vi "AmmeterComm.vi"() -> ()   [LabVIEW 2010]
uses:
  VarableID.ctl
  AmmeterGlobalCostants.vi
panel:
  out "display":T1={"电压/V"=[220.633378, 0.0, 0.0, 0.0, 0.0, 0.0, 0.0, 0.0], "测量变量显示"={"number: 0 to 1"=0.0, "number: 0 to 1"=0.0, "number: 0 to 1"=0.0}, "测量变量显示 2"={"number: 0 to 1"=0.0, "number: 0 to 1"=0.0, "number: 0 to 1"=0.0}}
  in  "视在功率":bool=TRUE
  in  "功率因数":bool=TRUE
  in  "电压":bool=TRUE
  in  "电流":bool=TRUE
  in  "退出系统":bool
  in  "软件使用说明":bool
  in  "启动采集":bool=TRUE
  # "CPES能源信息采集系统"
  # "信号采集选项"
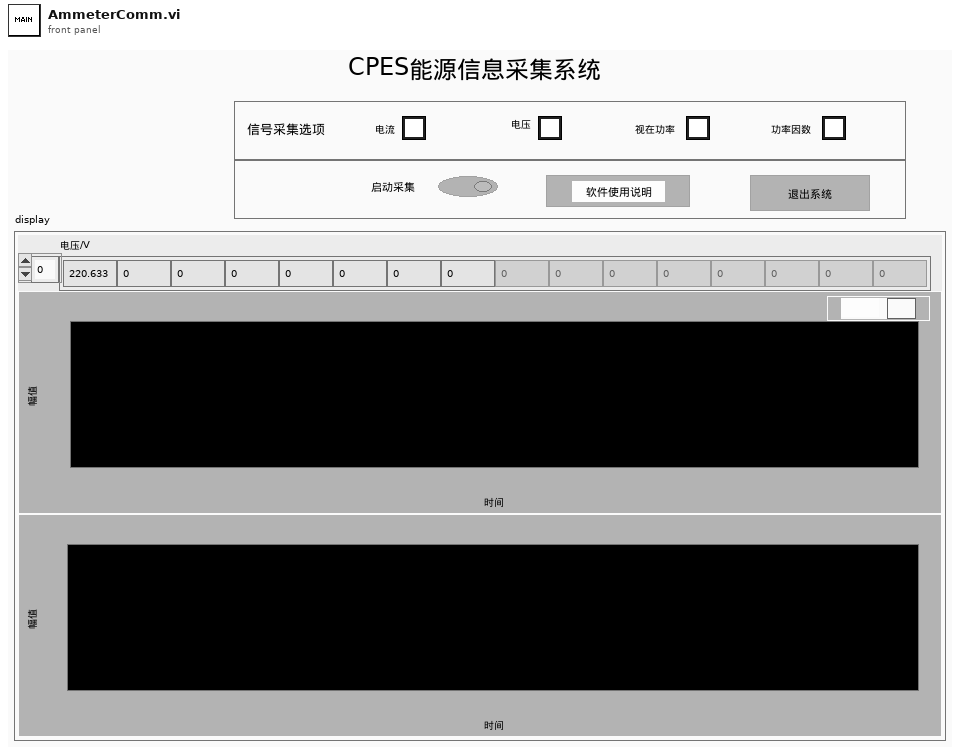
[diagram p1: front panel]
types:
  T1 = cluster{"电压/V":dbl[], "测量变量显示":cluster{"number: 0 to 1":dbl, "number: 0 to 1":dbl, "number: 0 to 1":dbl}, "测量变量显示 2":cluster{"number: 0 to 1":dbl, "number: 0 to 1":dbl, "number: 0 to 1":dbl}}
  T2 = cluster{"测量变量显示":refnum<vi>, "测量变量显示 2":refnum<vi>, "电压/V":refnum<vi>}
  T3 = typedef "OutputDataFormat.ctl" = cluster{"property":string, "dataIdentity":string, "value":string, "address":string, "timeStamp":string, "unit":string, "numID":i32, "VarableID":T4}
  T4 = typedef "VarableID.ctl" = enum16{"current", "power", "PF", "voltage"}
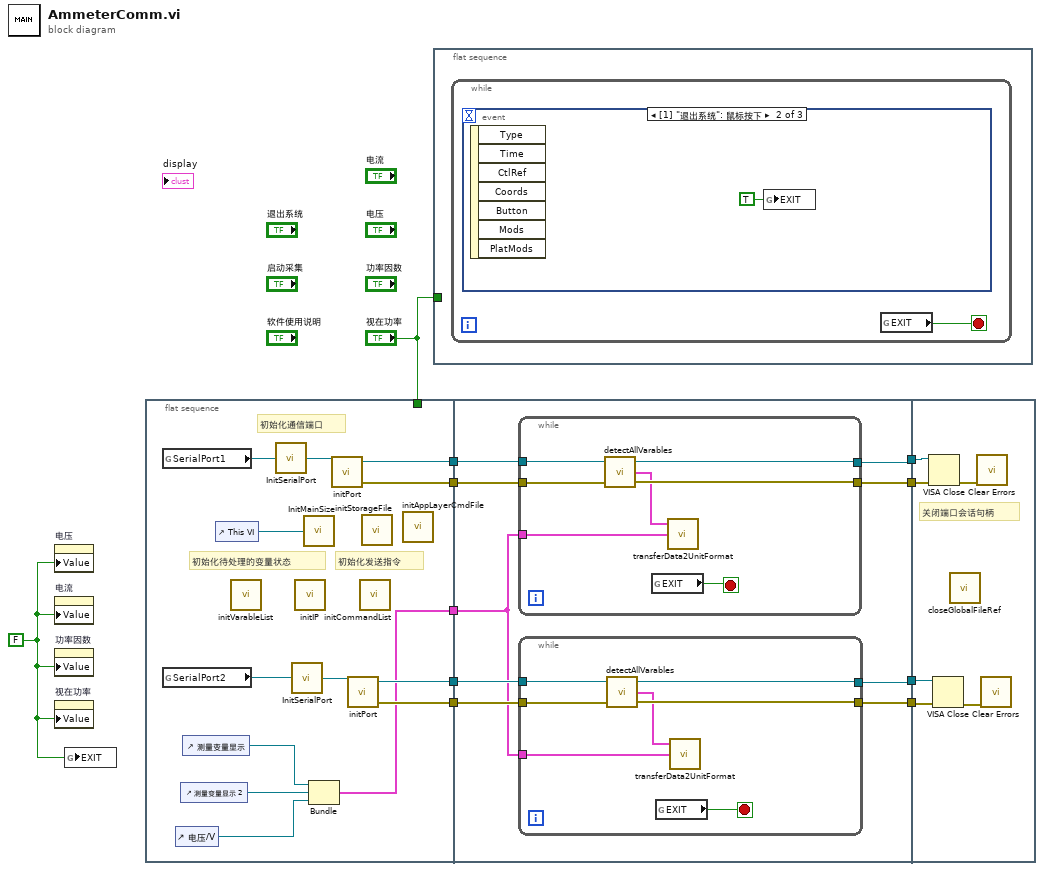
[diagram p0: block diagram]
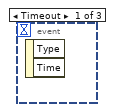
[diagram p2: hidden frame]
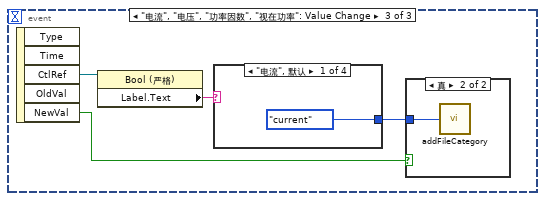
[diagram p3: hidden frame]
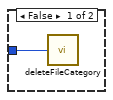
[diagram p4: hidden frame]
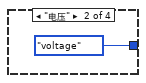
[diagram p5: hidden frame]
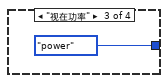
[diagram p6: hidden frame]
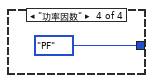
[diagram p7: hidden frame]
diagram:
  w1 = FALSE
  n1 = property on="电压" class="Bool (严格)"("Value"=w1) -> ()  [unwired: 2 in, 2 out]
  n2 = property on="电流" class="Bool (严格)"("Value"=w1) -> ()  [unwired: 2 in, 2 out]
  n3 = property on="功率因数" class="Bool (严格)"("Value"=w1) -> ()  [unwired: 2 in, 2 out]
  n4 = property on="视在功率" class="Bool (严格)"("Value"=w1) -> ()  [unwired: 2 in, 2 out]
  n5 = global write "AmmeterGlobalCostants.vi" "EXIT"(w1) -> ()
  n6 = flat-sequence {
    tunnel: [w23] -> w5
    tunnel: "视在功率" -> [_]
    tunnel: [w24] -> w6
    tunnel: [w19] -> w4
    tunnel: [w18] -> w3
    tunnel: [w14] -> w2
    tunnel: w6 -> [w33]
    tunnel: [w32] -> w11
    tunnel: [w31] -> w10
    tunnel: w5 -> [w30]
    tunnel: w4 -> [w29]
    tunnel: w3 -> [w28]
    tunnel: [w27] -> w8
    tunnel: [w26] -> w7
    tunnel: w2 -> [w25]
    tunnel: w11 -> [w53]
    tunnel: w10 -> [w52]
    tunnel: w8 -> [w51]
    tunnel: w7 -> [w50]
    frame #0 {
      # "初始化发送指令"
      # "初始化通信端口"
      # "初始化待处理的变量状态"
      n7 = global read "AmmeterGlobalCostants.vi" "SerialPort1"() -> (w17:refnum<visa-resource-name>)
      n8 = global read "AmmeterGlobalCostants.vi" "SerialPort2"() -> (w16:refnum<visa-resource-name>)
      n9 = control-ref of="电压/V"() -> (w15:refnum<vi>)
      n10 = control-ref of="测量变量显示 2"() -> (w13:refnum<vi>)
      n11 = control-ref of="测量变量显示"() -> (w12:refnum<vi>)
      n12 = control-ref of="This VI"() -> (w21:refnum<vi>)
      n13 = call "initVarableList.vi"() -> ()  [unwired: 12 in]
      n14 = call "InitSerialPort.vi"("default resource name"=w17) -> ("VISA resource name out"=w22:refnum<visa-resource-name>)
      n15 = call "InitSerialPort.vi"("default resource name"=w16) -> ("VISA resource name out"=w20:refnum<visa-resource-name>)
      n16 = call "initIP.vi"() -> ()  [unwired: 12 in]
      n17 = call "InitMainSize.vi"("VI Refnum In"=w21) -> ()  [unwired: 1 out]
      n18 = Bundle("测量变量显示"=w12, "测量变量显示 2"=w13, "电压/V"=w15) -> (w14:T2)  [unwired: 1 in]
      n19 = call "initPort.vi"("VISA resource name"=w22) -> ("error out"=w24:errorcluster, "reference out"=w23:refnum<visa-resource-name>)  [unwired: 3 in]
      n20 = call "initPort.vi"("VISA resource name"=w20) -> ("error out"=w18:errorcluster, "reference out"=w19:refnum<visa-resource-name>)  [unwired: 3 in]
      n21 = call "initCommandList.vi"() -> ()  [unwired: 12 in]
      n22 = call "initStorageFile.vi"() -> ()  [unwired: 12 in]
      n23 = call "initAppLayerCmdFile.vi"() -> ()  [unwired: 12 in]
    }
    frame #1 {
      n24 = while {
        tunnel: w33 -> [w44]
        tunnel: [w45] -> w32
        tunnel: [w47] -> w31
        tunnel: w30 -> [w46]
        tunnel: w25 -> [w41]
        stop <- w42 stop-if-true
        n25 = call "detectAllVarables.vi"("error in (no error)"=w44, "VISA resource name"=w46) -> ("error out"=w47:errorcluster, "Data"=w43:T3[], "VISA resource name 2"=w45:refnum<visa-resource-name>)  [unwired: 1 in]
        n26 = global read "AmmeterGlobalCostants.vi" "EXIT"() -> (w42:bool)
        n27 = call "transferData2UnitFormat.vi"("displayRef"=w41, "Data"=w43) -> ()  [unwired: 3 in, 1 out]
      }
      n28 = while {
        tunnel: w28 -> [w37]
        tunnel: [w38] -> w27
        tunnel: [w40] -> w26
        tunnel: w29 -> [w39]
        tunnel: w25 -> [w34]
        stop <- w35 stop-if-true
        n29 = call "detectAllVarables.vi"("error in (no error)"=w37, "VISA resource name"=w39) -> ("error out"=w40:errorcluster, "Data"=w36:T3[], "VISA resource name 2"=w38:refnum<visa-resource-name>)  [unwired: 1 in]
        n30 = global read "AmmeterGlobalCostants.vi" "EXIT"() -> (w35:bool)
        n31 = call "transferData2UnitFormat.vi"("displayRef"=w34, "Data"=w36) -> ()  [unwired: 3 in, 1 out]
      }
    }
    frame #2 {
      # "关闭端口会话句柄"
      n32 = VISA Close(VISA resource name=w53, error in (no error)=w52) -> (error out=w49:errorcluster)
      n33 = VISA Close(VISA resource name=w51, error in (no error)=w50) -> (error out=w48:errorcluster)
      n34 = call "closeGlobalFileRef.vi"() -> ()  [unwired: 12 in]
      n35 = call <vilib>:"Clear Errors.vi"("error in (no error)"=w49) -> ()  [unwired: 6 in, 1 out]
      n36 = call <vilib>:"Clear Errors.vi"("error in (no error)"=w48) -> ()  [unwired: 6 in, 1 out]
    }
  }
  n37 = flat-sequence {
    tunnel: "视在功率" -> [_]
    frame #0 {
      n38 = while {
        stop <- w54 stop-if-true
        n39 = event shown="[1] \"退出系统\": 鼠标按下" {
          selector: _ -> [_ _ _]
          dyn-events: _ -> [_ _ _]
          timeout: _ -> [_ _ _]
          event Timeout {
            n40 = event-data() -> ()  [unwired: 1 in, 2 out]
          }
          event "退出系统": Mouse Down {
            n41 = event-data() -> ()  [unwired: 1 in, 7 out]
            n42 = global write "AmmeterGlobalCostants.vi" "EXIT"(TRUE ("EXIT")) -> ()
          }
          event "电流", "电压", "功率因数", "视在功率": Value Change {
            n43 = event-data() -> ("CtlRef"=w56:refnum<vi>, "NewVal"=w57:bool)  [unwired: 1 in, 3 out]
            n44 = property class="Bool (严格)"(reference=w56) -> ("Label.Text"=w59:string)  [unwired: 1 in, 2 out]
            n45 = case shown="\"电流\", 默认" w59 {
              tunnel: [VarableID."current" ("VarableID") VarableID."voltage" ("VarableID") VarableID."power" ("VarableID") VarableID."PF" ("VarableID")] -> w58
              frame "电流", Default {
              }
              frame "电压" {
              }
              frame "视在功率" {
              }
              frame "功率因数" {
              }
            }
            n46 = case shown="真" w57 {
              tunnel: w58 -> [w60 w61]
              frame False {
                n47 = call "deleteFileCategory.vi"("VarableID"=w60) -> ()  [unwired: 1 in]
              }
              frame True {
                n48 = call "addFileCategory.vi"("VarableID"=w61) -> ()  [unwired: 1 in]
              }
            }
          }
        }
        n49 = global read "AmmeterGlobalCostants.vi" "EXIT"() -> (w54:bool)
      }
    }
  }
